vi "HRM-init_main.vi"() -> (0 "error out":errorcluster, 3 "Init cluster":T1)   [LabVIEW 2020]
uses:
  HRM-init_cluster.ctl
  HRM-User_events.ctl
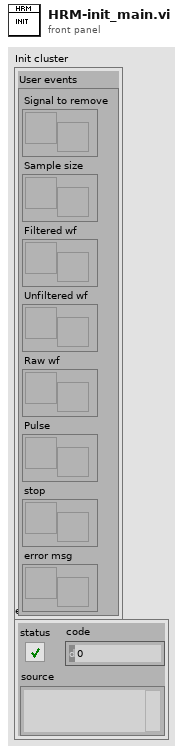
[diagram p1: front panel]
types:
  T1 = typedef "HRM-init_cluster.ctl" = cluster{"User events":T2}
  T2 = typedef "HRM-User_events.ctl" = cluster{"Signal to remove":refnum<user-event>, "Sample size":refnum<user-event>, "Filtered wf":refnum<user-event>, "Unfiltered wf":refnum<user-event>, "Raw wf":refnum<user-event>, "Pulse":refnum<user-event>, "stop":refnum<user-event>, "error msg":refnum<user-event>}
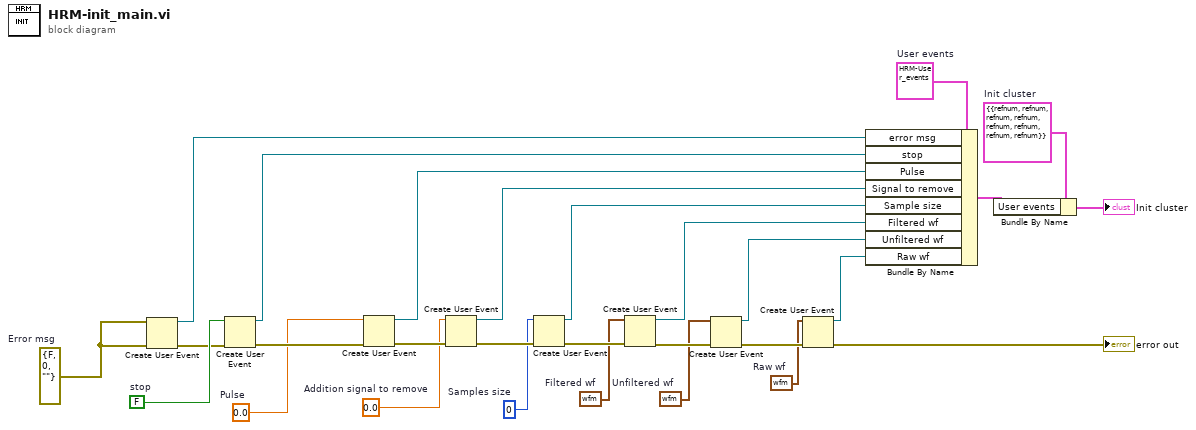
[diagram p0: block diagram]
diagram:
  w2 = errorcluster {"status"=FALSE, "code"=0, "source"=""}  # Error msg
  w24 = FALSE  # stop
  w22 = T1 {"User events"={"Signal to remove"=refnum, "Sample size"=refnum, "Filtered wf"=refnum, "Unfiltered wf"=refnum, "Raw wf"=refnum, "Pulse"=refnum, "stop"=refnum, "error msg"=refnum}}  # Init cluster
  w19 = 0.0  # Pulse
  w13 = T2 {"Signal to remove"=refnum, "Sample size"=refnum, "Filtered wf"=refnum, "Unfiltered wf"=refnum, "Raw wf"=refnum, "Pulse"=refnum, "stop"=refnum, "error msg"=refnum}  # User events
  w8 = 0  # Samples size
  w7 = 0.0  # Addition signal to remove
  w6 = waveform(dbl) {"t0"=timestamp(0 s since 1904-01-01), "dt"=1.0, "Y"=[]}  # Filtered wf
  w5 = waveform(dbl) {"t0"=timestamp(0 s since 1904-01-01), "dt"=1.0, "Y"=[]}  # Unfiltered wf
  w4 = waveform(dbl) {"t0"=timestamp(0 s since 1904-01-01), "dt"=1.0, "Y"=[]}  # Raw wf
  n1 = Create User Event(user event datatype=w2, error in=w2) -> (user event=w1:refnum<user-event>, error out=w3:errorcluster)
  n2 = Create User Event(user event datatype=w24, error in=w3) -> (user event=w26:refnum<user-event>, error out=w25:errorcluster)
  n3 = Create User Event(user event datatype=w19, error in=w25) -> (user event=w20:refnum<user-event>, error out=w21:errorcluster)
  n4 = Create User Event(user event datatype=w7, error in=w21) -> (user event=w14:refnum<user-event>, error out=w12:errorcluster)
  n5 = Create User Event(user event datatype=w8, error in=w12) -> (user event=w15:refnum<user-event>, error out=w11:errorcluster)
  n6 = Create User Event(user event datatype=w6, error in=w11) -> (user event=w16:refnum<user-event>, error out=w10:errorcluster)
  n7 = Create User Event(user event datatype=w5, error in=w10) -> (user event=w17:refnum<user-event>, error out=w9:errorcluster)
  n8 = Create User Event(user event datatype=w4, error in=w9) -> (user event=w18:refnum<user-event>, error out=→"error out":errorcluster)
  n9 = Bundle By Name(cluster=w13, "error msg"=w1, "stop"=w26, "Pulse"=w20, "Signal to remove"=w14, "Sample size"=w15, "Filtered wf"=w16, "Unfiltered wf"=w17, "Raw wf"=w18) -> (w23:T2)
  n10 = Bundle By Name(cluster=w22, "User events"=w23) -> (→"Init cluster":T1)
